vi "Google Map (Keith Koch's conflicted copy 2013-05-10).vi"   [LabVIEW 2011]
uses:
  _GlobalVariables&Libraries/ATV Program Global Variables.vi
types:
  T1 = cluster{"X":dbl, "Y":dbl, "Zoom":sgl, "Map Type":string, "Google Maps API Key":string, "Map Refresh Rate (ms)":u32, "Navigation Path Color":u32, "Navigation Path Weight":i32, "URL":string, "Boundary Coordinates":cluster{"Latitude":dbl, "Longitude":dbl}[], "GPS Balloon Character":string, "Boundary Path Color":u32, "Boundary Path Weight":i32, "GPS Balloon Size":string, "GPS Balloon Color":string, "GPS Path Color":u32, "GPS Path Weight":i32, "Disable Google Maps":bool}
  T2 = cluster{"End ATV Program":bool, "E-Stop":bool, "Save Logfile":bool, "Logfile Iteration Delay (ms)":u32, "Loop iteration time (ms)":u32, "Logfile Location":path, "Default GPS Navigation Path":path, "Computer":string, "Default GPS Boundary Path":path}
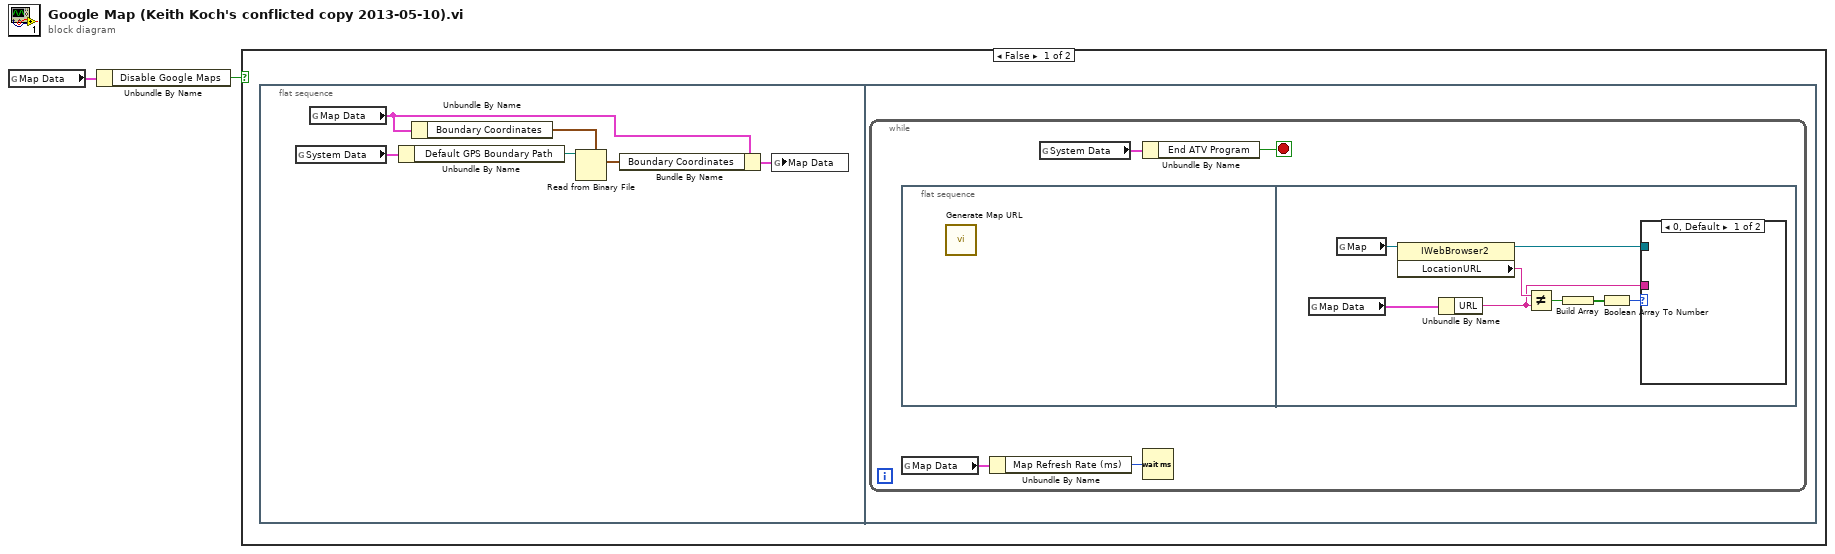
[diagram p0: block diagram]
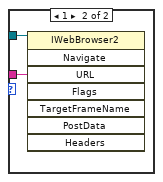
[diagram p2: hidden frame]
diagram:
  n1 = global read "ATV Program Global Variables.vi" "Map Data"() -> (w2:T1)
  n2 = Unbundle By Name(w2) -> ("Disable Google Maps"=w1:bool)
  n3 = case shown="False" w1 {
    frame False {
      n4 = flat-sequence {
        frame #0 {
          n5 = global read "ATV Program Global Variables.vi" "System Data"() -> (w3:T2)
          n6 = global read "ATV Program Global Variables.vi" "Map Data"() -> (w7:T1)
          n7 = Unbundle By Name(w3) -> ("Default GPS Boundary Path"=w8:path)
          n8 = Unbundle By Name(w7) -> ("Boundary Coordinates"=w6:cluster{"Latitude":dbl, "Longitude":dbl}[])
          n9 = Read from Binary File(5:w6, 11:w8) -> (2:w4:cluster{"Latitude":dbl, "Longitude":dbl}[])  [unwired: 4 in, 3 out]
          n10 = Bundle By Name(cluster=w7, "Boundary Coordinates"=w4) -> (w5:T1)
          n11 = global write "ATV Program Global Variables.vi" "Map Data"(w5) -> ()
        }
        frame #1 {
          n12 = while {
            stop <- w10 stop-if-true
            n13 = flat-sequence {
              frame #0 {
                n14 = call "Generate Map URL.vi"() -> ()  [unwired: 12 in]
              }
              frame #1 {
                n15 = global read "ATV Program Global Variables.vi" "Map Data"() -> (w14:T1)
                n16 = global read "ATV Program Global Variables.vi" "Map"() -> (w15:refnum<k7>)
                n17 = property class="IWebBrowser2"(reference=w15) -> (reference out=w20:refnum<k7>, "LocationURL"=w18:string)  [unwired: 1 in, 1 out]
                n18 = Unbundle By Name(w14) -> ("URL"=w13:string)
                n19 = Not Equal?(x=w18, y=w13) -> (x != y?=w19:bool)
                n20 = Build Array(w19) -> (w17:bool[])
                n21 = Boolean Array To Number(Boolean array=w17) -> (number=w16:u32)
                n22 = case shown="0, Default" w16 {
                  tunnel: w13 -> [_ w22]
                  tunnel: w20 -> [_ w21]
                  frame 0, Default {
                  }
                  frame 1 {
                    n23 = invoke class="IWebBrowser2" method="Navigate"(reference=w21, "URL"=w22) -> ()  [unwired: 6 in, 8 out]
                  }
                }
              }
            }
            n24 = global read "ATV Program Global Variables.vi" "Map Data"() -> (w12:T1)
            n25 = Unbundle By Name(w12) -> ("Map Refresh Rate (ms)"=w9:u32)
            n26 = global read "ATV Program Global Variables.vi" "System Data"() -> (w11:T2)
            n27 = Unbundle By Name(w11) -> ("End ATV Program"=w10:bool)
            n28 = Wait (ms)(milliseconds to wait=w9) -> ()  [unwired: 1 out]
          }
        }
      }
    }
    frame True {
    }
  }
